vi "RVTBOX SampleCode_MultPort.vi"(11 "Modbus TCP Setting":T4={"TCP address"="192.168.178.2", "CH"=enum."Port1", "Sample Rate"=7812, "Port"=502}) -> ()   [LabVIEW 2022 SP3]
uses:
  Ctl/TCP Setting.ctl
  Ctl/Modbus Function TCP.ctl
  PortStatus.ctl
  E:/RVT_CONTROLBOX/RVT BOX SampleCode/LabVIEW/BOX SampleCode/DLL/Modbus.dll
  DLL/Modbus.dll
panel:
  in  "ON (Port1 ~ Port4) 2":bool[](array[boolean])=[TRUE, TRUE, FALSE, FALSE]
  out "Data Length 抓資料後的剩餘長度 2":u16(graph)=22989
  out "Waveform Chart 2":dbl[][](graph)=[[-0.00146484375, 0.0020751953125, -0.00146484375], [-0.000732421875, 0.001953125, -0.00048828125], [-0.00048828125, 0.000732421875, 0.0001220703125], [-0.001220703125, 0.0, 0.00048828125], [-0.002197265625, 0.001220703125, 0.0006103515625], [-0.002685546875, 0.0025634765625, 0.000732421875], [-0.0023193359375, 0.0018310546875, 0.0010986328125], [-0.0015869140625, 0.000732421875, 0.001708984375], [-0.001220703125, 0.000732421875, 0.002197265625], [-0.0018310546875, 0.0006103515625, 0.0020751953125], [-0.00244140625, -0.0003662109375, 0.0020751953125], [-0.0023193359375, -0.0006103515625, 0.0025634765625], [-0.002197265625, 0.00048828125, 0.0025634765625], [-0.0023193359375, 0.0009765625, 0.001953125], [-0.002197265625, 0.0003662109375, 0.0015869140625], [-0.0013427734375, 0.0003662109375, 0.0018310546875], [-0.0001220703125, 0.0006103515625, 0.0020751953125], [0.00048828125, 0.0001220703125, 0.0020751953125], [0.00048828125, 0.0, 0.001708984375], [0.0001220703125, 0.0009765625, 0.0013427734375], [0.0, 0.001708984375, 0.0010986328125], [-0.0001220703125, 0.0009765625, 0.0006103515625], [-0.0003662109375, 0.0, 0.0], [-0.0003662109375, 0.0, 0.0], [0.0, 0.0, 0.00048828125], [0.0003662109375, -0.00048828125, 0.00048828125], [0.0006103515625, -0.0009765625, 0.0001220703125], [0.0008544921875, -0.0006103515625, 0.000732421875], [0.000732421875, 0.0006103515625, 0.001708984375], [0.0003662109375, 0.002197265625, 0.0013427734375], [0.0001220703125, 0.003173828125, -0.000244140625], [0.0, 0.0029296875, -0.0013427734375], [-0.0010986328125, 0.00146484375, -0.0009765625], [-0.00244140625, 0.00048828125, 0.00048828125], [-0.002685546875, 0.000732421875, 0.0013427734375], [-0.00244140625, 0.0015869140625, 0.0008544921875], [-0.0015869140625, 0.0015869140625, 0.0001220703125], [-0.0006103515625, 0.00048828125, 0.0008544921875], [-0.00048828125, 0.0, 0.00146484375], [-0.001708984375, 0.0006103515625, 0.00048828125], [-0.001953125, 0.0008544921875, -0.000732421875], [-0.0006103515625, 0.0, -0.0001220703125], [0.0, -0.0003662109375, 0.0009765625], [-0.001220703125, 0.0003662109375, 0.0009765625], [-0.001953125, 0.0008544921875, 0.00048828125], [-0.0006103515625, 0.0006103515625, 0.00146484375], [0.0003662109375, 0.0006103515625, 0.003173828125], [-0.0003662109375, 0.0010986328125, 0.003662109375], [-0.001220703125, 0.0013427734375, 0.00244140625], [-0.001220703125, 0.0009765625, 0.00146484375], [-0.001708984375, 0.0, 0.001953125], [-0.002685546875, -0.001220703125, 0.00244140625], [-0.0029296875, -0.0010986328125, 0.0015869140625], [-0.0023193359375, 0.00048828125, 0.0003662109375], [-0.001708984375, 0.0013427734375, 0.000244140625], [-0.0010986328125, 0.0003662109375, 0.0009765625], [-0.0009765625, -0.000732421875, 0.0015869140625], [-0.001220703125, -0.0003662109375, 0.001708984375], [-0.000732421875, 0.0001220703125, 0.0006103515625], [-0.0001220703125, 0.0, -0.0009765625], [-0.00048828125, -0.00048828125, -0.0009765625], [-0.001220703125, -0.0003662109375, 0.0010986328125], [-0.000732421875, 0.0, 0.0025634765625], [0.0003662109375, 0.0003662109375, 0.0013427734375], [0.0010986328125, 0.000732421875, 0.0], [0.0013427734375, 0.0006103515625, 0.0], [0.0009765625, 0.00048828125, 0.0], [0.0, 0.0009765625, -0.0008544921875], [-0.0010986328125, 0.0018310546875, -0.001220703125], [-0.001708984375, 0.00146484375, -0.000244140625], [-0.0020751953125, 0.0001220703125, 0.0003662109375], [-0.0025634765625, -0.0001220703125, 0.00048828125], [-0.002197265625, 0.0003662109375, 0.00048828125], [-0.0010986328125, 0.000244140625, 0.000244140625], [-0.0003662109375, -0.0003662109375, -0.00048828125], [-0.000244140625, -0.0003662109375, -0.0010986328125], [-0.000244140625, 0.00048828125, -0.0009765625], [0.0, 0.0006103515625, -0.0009765625], [0.00048828125, 0.0, -0.0010986328125], [0.0008544921875, -0.0006103515625, -0.0001220703125], [0.0006103515625, -0.000732421875, 0.001220703125], [-0.0001220703125, -0.0010986328125, 0.001220703125], [-0.000732421875, -0.0006103515625, -0.0003662109375], [-0.0006103515625, 0.0008544921875, -0.0018310546875], [-0.0008544921875, 0.001953125, -0.001953125], [-0.0018310546875, 0.0015869140625, -0.001708984375], [-0.0025634765625, 0.000244140625, -0.0013427734375], [-0.002197265625, -0.0006103515625, -0.000732421875], [-0.0015869140625, -0.00146484375, 0.0], [-0.00146484375, -0.001708984375, 0.0006103515625], [-0.001220703125, -0.0010986328125, 0.0018310546875], [-0.0009765625, -0.0003662109375, 0.00244140625], [-0.001220703125, -0.0006103515625, 0.0013427734375], [-0.0018310546875, -0.0010986328125, 0.0], [-0.001953125, -0.000732421875, 0.0003662109375], [-0.001708984375, -0.0001220703125, 0.0018310546875], [-0.0018310546875, -0.0008544921875, 0.0020751953125], [-0.0015869140625, -0.001953125, 0.0010986328125], [-0.0003662109375, -0.001708984375, 0.0006103515625], [0.000244140625, -0.000244140625, 0.0008544921875], [-0.0003662109375, 0.000244140625, 0.0008544921875], [-0.0018310546875, -0.000244140625, 0.0001220703125], [-0.0020751953125, -0.000732421875, -0.0003662109375], [-0.0010986328125, -0.0003662109375, -0.000244140625], [-0.000244140625, 0.000244140625, 0.0], [-0.00048828125, 0.0, -0.000244140625], [-0.0010986328125, -0.0006103515625, -0.000732421875], [-0.0015869140625, -0.0009765625, -0.000244140625], [-0.001953125, -0.0006103515625, 0.0001220703125], [-0.0018310546875, -0.0003662109375, -0.000244140625], [-0.001220703125, -0.0003662109375, -0.000732421875], [-0.0009765625, -0.0001220703125, -0.0006103515625], [-0.0009765625, 0.0006103515625, -0.0006103515625], [-0.00048828125, 0.000732421875, -0.00048828125], [0.0006103515625, -0.000244140625, 0.000732421875], [0.0013427734375, -0.001220703125, 0.0015869140625], [0.0010986328125, -0.0006103515625, 0.0], [0.001220703125, 0.00048828125, -0.001953125], [0.001708984375, 0.0010986328125, -0.0018310546875], [0.000732421875, 0.0008544921875, -0.0008544921875], [-0.0015869140625, 0.0001220703125, -0.001220703125], [-0.003173828125, -0.0006103515625, -0.00146484375], [-0.0030517578125, -0.0006103515625, -0.000732421875], [-0.0023193359375, -0.000244140625, -0.000732421875], [-0.0015869140625, -0.001220703125, -0.0015869140625], [-0.000732421875, -0.0025634765625, -0.001220703125], [-0.0006103515625, -0.002197265625, 0.0], [-0.001220703125, -0.0008544921875, -0.0001220703125], [-0.0013427734375, -0.0006103515625, -0.000732421875], [-0.0003662109375, -0.0008544921875, -0.0003662109375], [0.0, 0.0, 0.0], [-0.0008544921875, 0.000732421875, -0.00048828125], [-0.001708984375, 0.0, -0.0006103515625], [-0.0018310546875, -0.0013427734375, 0.0001220703125], [-0.0015869140625, -0.001708984375, 0.0], [-0.000732421875, -0.00146484375, -0.0015869140625], [0.000244140625, -0.0015869140625, -0.001953125], [0.0003662109375, -0.0018310546875, -0.0008544921875], [-0.001220703125, -0.0018310546875, -0.0010986328125], [-0.0025634765625, -0.0013427734375, -0.00244140625], [-0.002197265625, -0.0010986328125, -0.0015869140625], [-0.0013427734375, -0.00146484375, 0.0008544921875], [-0.0018310546875, -0.0018310546875, 0.0013427734375], [-0.0020751953125, -0.0013427734375, -0.000244140625], [-0.0013427734375, -0.0006103515625, -0.0008544921875], [-0.0008544921875, -0.00048828125, 0.0], [-0.0008544921875, -0.00048828125, 0.0003662109375], [-0.000244140625, -0.0001220703125, -0.0001220703125], [0.000244140625, -0.00048828125, -0.00048828125], [-0.000244140625, -0.0015869140625, -0.000244140625], [-0.0006103515625, -0.00146484375, -0.0001220703125], [0.0001220703125, -0.000244140625, 0.0], [0.0008544921875, 0.0009765625, 0.0], [0.0006103515625, 0.0010986328125, 0.0003662109375], [0.0003662109375, 0.0001220703125, 0.000732421875], [0.0, -0.0009765625, 0.0009765625], [-0.000244140625, -0.0010986328125, 0.0009765625], [-0.0001220703125, 0.0, 0.0013427734375], [0.000732421875, 0.0, 0.0020751953125], [0.0006103515625, -0.001220703125, 0.001953125], [-0.0003662109375, -0.0020751953125, 0.0009765625], [-0.000732421875, -0.0009765625, 0.00048828125], [-0.0003662109375, 0.000244140625, 0.00146484375], [-0.000244140625, 0.000244140625, 0.00244140625], [-0.000244140625, -0.0003662109375, 0.001953125], [0.0001220703125, -0.0003662109375, 0.0013427734375], [0.000732421875, 0.0, 0.001708984375], [0.0013427734375, -0.000244140625, 0.00244140625], [0.0023193359375, -0.001220703125, 0.0028076171875], [0.001953125, -0.0010986328125, 0.0030517578125], [0.0, 0.0001220703125, 0.003173828125], [-0.001708984375, 0.0003662109375, 0.0028076171875], [-0.00146484375, -0.0010986328125, 0.00146484375], [-0.0008544921875, -0.001953125, 0.000244140625], [-0.00146484375, -0.00048828125, 0.0], [-0.00146484375, 0.000732421875, 0.0006103515625], [0.0001220703125, 0.00048828125, 0.0009765625], [0.001708984375, 0.00048828125, 0.0001220703125], [0.00146484375, 0.0013427734375, -0.00048828125], [0.0006103515625, 0.00146484375, 0.0003662109375], [0.0003662109375, 0.000244140625, 0.001953125], [-0.0001220703125, -0.0010986328125, 0.00146484375], [-0.00146484375, -0.002197265625, 0.0], [-0.001953125, -0.00244140625, -0.0001220703125], [-0.0008544921875, -0.0015869140625, 0.0008544921875], [0.000732421875, 0.0, 0.000732421875], [0.0018310546875, 0.0010986328125, -0.000244140625], [0.0023193359375, 0.000732421875, -0.000244140625], [0.00244140625, 0.0, 0.0003662109375], [0.002197265625, -0.0006103515625, 0.0], [0.0009765625, -0.001220703125, -0.0006103515625], [-0.001220703125, -0.001708984375, 0.0], [-0.0029296875, -0.001220703125, 0.0013427734375], [-0.002685546875, -0.0006103515625, 0.001708984375], [-0.0008544921875, -0.0009765625, 0.001220703125], [0.0006103515625, -0.00146484375, 0.000732421875], [0.001220703125, -0.000732421875, 0.0003662109375], [0.00146484375, 0.0006103515625, 0.0001220703125], [0.0009765625, 0.0006103515625, 0.000244140625], [0.0, -0.000244140625, 0.000244140625], [-0.0009765625, -0.0003662109375, 0.0], [-0.0010986328125, -0.00048828125, -0.0001220703125], [-0.0009765625, -0.0013427734375, -0.0001220703125], [-0.00146484375, -0.001708984375, 0.0006103515625], [-0.0015869140625, -0.0006103515625, 0.0020751953125], [-0.000732421875, 0.0003662109375, 0.0023193359375], [0.00048828125, 0.0, 0.000732421875], [0.0010986328125, -0.0001220703125, -0.0003662109375], [0.0009765625, -0.0001220703125, 0.000244140625], [0.0001220703125, -0.0008544921875, 0.0015869140625], [-0.0006103515625, -0.0015869140625, 0.001953125], [-0.0008544921875, -0.0015869140625, 0.001708984375], [-0.0003662109375, -0.001220703125, 0.001953125], [-0.0001220703125, -0.00048828125, 0.0020751953125], [0.0, 0.0003662109375, 0.0009765625], [0.00048828125, 0.0006103515625, -0.000244140625], [0.0008544921875, 0.0, -0.000244140625], [0.0008544921875, -0.0001220703125, 0.000244140625], [0.0010986328125, 0.0001220703125, 0.0], [0.001708984375, -0.0001220703125, -0.0006103515625], [0.00146484375, -0.0010986328125, -0.000244140625], [0.0001220703125, -0.0020751953125, 0.0006103515625], [-0.0010986328125, -0.0028076171875, 0.0006103515625], [-0.0018310546875, -0.002197265625, -0.0001220703125], [-0.0018310546875, 0.0, -0.0003662109375], [-0.0013427734375, 0.0008544921875, 0.0003662109375], [-0.00048828125, 0.0001220703125, 0.001220703125], [0.0, 0.0, 0.0010986328125], [-0.0001220703125, 0.0010986328125, 0.0003662109375], [0.0, 0.0015869140625, -0.0001220703125], [0.00048828125, 0.0013427734375, -0.0006103515625], [0.000732421875, 0.0010986328125, -0.0015869140625], [0.0, 0.00048828125, -0.0020751953125], [-0.00048828125, -0.0001220703125, -0.001220703125], [0.0, 0.0, -0.000244140625], [0.0015869140625, 0.0003662109375, -0.000244140625], [0.0029296875, 0.0001220703125, -0.0006103515625], [0.0025634765625, 0.0001220703125, 0.0], [0.00146484375, 0.00146484375, 0.00048828125], [0.0015869140625, 0.001953125, -0.0003662109375], [0.0018310546875, 0.000732421875, -0.0008544921875], [0.0, -0.0003662109375, -0.0001220703125], [-0.002685546875, -0.000244140625, 0.0], [-0.0035400390625, 0.000244140625, -0.0015869140625], [-0.001708984375, 0.00048828125, -0.002197265625], [-0.0001220703125, 0.00048828125, -0.001220703125], [0.0, 0.0006103515625, -0.0009765625], [0.0003662109375, 0.001220703125, -0.0013427734375], [0.0013427734375, 0.00146484375, -0.0009765625], [0.0013427734375, 0.0003662109375, -0.0001220703125], [0.0006103515625, -0.001220703125, 0.0], [0.0, -0.0018310546875, -0.00048828125], [-0.0006103515625, -0.001708984375, -0.0009765625], [-0.00146484375, -0.0013427734375, -0.001220703125], [-0.00146484375, -0.0010986328125, -0.000732421875], [-0.0003662109375, -0.00048828125, 0.0009765625], [0.0006103515625, 0.000244140625, 0.002197265625], [0.001220703125, 0.000732421875, 0.001953125], [0.0020751953125, 0.0003662109375, 0.001220703125], [0.0025634765625, -0.0003662109375, 0.001220703125], [0.00146484375, -0.0009765625, 0.0009765625], [-0.0008544921875, -0.00146484375, -0.0003662109375], [-0.0028076171875, -0.0020751953125, -0.0020751953125], [-0.0029296875, -0.0020751953125, -0.001953125], [-0.0020751953125, -0.000732421875, -0.000244140625], [-0.0006103515625, 0.000244140625, 0.0006103515625], [0.0009765625, 0.00048828125, -0.0001220703125], [0.0023193359375, 0.0008544921875, -0.00146484375], [0.002685546875, 0.001708984375, -0.0008544921875], [0.001953125, 0.001708984375, 0.00146484375], [0.0008544921875, 0.0009765625, 0.0032958984375], [0.00048828125, 0.0, 0.00244140625], [0.0, -0.0008544921875, 0.0], [-0.0008544921875, -0.0010986328125, -0.0018310546875], [-0.0008544921875, 0.000244140625, -0.001708984375], [0.00048828125, 0.001220703125, -0.0010986328125], [0.001220703125, 0.000244140625, -0.000732421875], [0.0, -0.00048828125, -0.000732421875], [-0.0003662109375, 0.0003662109375, -0.0008544921875], [0.0008544921875, 0.00146484375, -0.0006103515625], [0.001220703125, 0.00048828125, 0.0001220703125], [-0.00048828125, -0.0001220703125, 0.0009765625], [-0.001953125, 0.000732421875, 0.00048828125], [-0.00146484375, 0.0018310546875, -0.000732421875], [-0.0006103515625, 0.0015869140625, -0.00146484375], [-0.0008544921875, 0.000732421875, -0.001220703125], [-0.0010986328125, 0.0003662109375, -0.0006103515625], [-0.00048828125, 0.000732421875, -0.0001220703125], [0.000244140625, 0.0010986328125, 0.0001220703125], [0.0009765625, 0.000244140625, 0.0], [0.001708984375, -0.001220703125, -0.000244140625], [0.0015869140625, -0.0018310546875, 0.0], [0.0, -0.001220703125, 0.0006103515625], [-0.001708984375, -0.0006103515625, 0.00048828125], [-0.0013427734375, 0.0, -0.000732421875], [0.000244140625, 0.000732421875, -0.0010986328125], [0.0009765625, 0.0013427734375, 0.0006103515625], [0.0001220703125, 0.0010986328125, 0.0020751953125], [-0.0003662109375, 0.0010986328125, 0.0009765625], [0.0001220703125, 0.0010986328125, 0.0], [0.0010986328125, 0.00048828125, 0.0009765625], [0.0010986328125, -0.000244140625, 0.0018310546875], [0.0, -0.0006103515625, 0.0009765625], [-0.0009765625, -0.00048828125, 0.0003662109375], [-0.0008544921875, 0.0001220703125, 0.000732421875], [-0.0006103515625, 0.00146484375, 0.000732421875], [-0.0009765625, 0.0025634765625, 0.0006103515625], [-0.0009765625, 0.00244140625, 0.0010986328125], [-0.0003662109375, 0.001708984375, 0.0006103515625], [0.000244140625, 0.0010986328125, -0.0006103515625], [0.0009765625, 0.00048828125, -0.000732421875], [0.0018310546875, -0.0001220703125, -0.0001220703125], [0.0018310546875, -0.00048828125, -0.0003662109375], [0.0006103515625, -0.000244140625, 0.0], [-0.0008544921875, 0.0, 0.00146484375], [-0.0015869140625, 0.00048828125, 0.0018310546875], [-0.001220703125, 0.0015869140625, 0.0008544921875], [-0.00048828125, 0.00244140625, 0.0006103515625], [0.0001220703125, 0.0020751953125, 0.000732421875], [0.00048828125, 0.0006103515625, 0.0], [0.000732421875, 0.0, -0.000244140625], [0.0008544921875, 0.000244140625, 0.0006103515625], [0.000244140625, 0.000732421875, 0.00048828125], [-0.0010986328125, 0.000732421875, -0.0006103515625], [-0.0025634765625, 0.0006103515625, -0.0009765625], [-0.00341796875, 0.0009765625, -0.0006103515625], [-0.003173828125, 0.001708984375, -0.0008544921875], [-0.002197265625, 0.0020751953125, -0.00048828125], [-0.0010986328125, 0.001220703125, 0.0003662109375], [-0.000244140625, 0.0003662109375, 0.00048828125], [0.0, 0.00048828125, 0.0], [-0.001220703125, 0.0006103515625, -0.000244140625], [-0.00244140625, 0.0003662109375, -0.0001220703125], [-0.001708984375, 0.0003662109375, 0.0003662109375], [-0.0003662109375, 0.0006103515625, 0.001220703125], [-0.00048828125, 0.000732421875, 0.001708984375], [-0.001708984375, 0.000732421875, 0.0006103515625], [-0.00146484375, 0.0008544921875, -0.00048828125], [0.0, 0.000732421875, 0.0001220703125], [0.001220703125, 0.0006103515625, 0.002197265625], [0.0013427734375, 0.0010986328125, 0.002685546875], [0.000732421875, 0.00146484375, 0.00146484375], [-0.00048828125, 0.0006103515625, 0.0009765625], [-0.001708984375, 0.0, 0.0020751953125], [-0.002197265625, 0.000244140625, 0.002197265625], [-0.0015869140625, 0.0006103515625, 0.0006103515625], [-0.00048828125, 0.0, 0.0], [0.0001220703125, -0.00048828125, 0.0013427734375], [0.0001220703125, 0.0001220703125, 0.002197265625], [0.0, 0.0009765625, 0.001220703125], [0.00048828125, 0.0008544921875, 0.0008544921875], [0.001220703125, 0.0, 0.001708984375], [0.0009765625, -0.0009765625, 0.0015869140625], [0.0, -0.0010986328125, 0.0001220703125], [-0.000732421875, -0.0008544921875, -0.0003662109375], [-0.0009765625, -0.0009765625, 0.0], [-0.001220703125, -0.0010986328125, -0.0003662109375], [-0.0015869140625, 0.0001220703125, -0.001220703125], [-0.0015869140625, 0.0020751953125, -0.0009765625], [-0.0010986328125, 0.0029296875, 0.0], [-0.0003662109375, 0.0023193359375, 0.0], [0.0, 0.0020751953125, -0.00048828125], [0.000244140625, 0.002685546875, -0.0008544921875], [0.0010986328125, 0.0025634765625, -0.001220703125], [0.0010986328125, 0.0008544921875, -0.0023193359375], [0.0, -0.0003662109375, -0.0029296875], [-0.0013427734375, 0.0, -0.0018310546875], [-0.001953125, 0.0006103515625, 0.0], [-0.001953125, 0.00048828125, 0.0006103515625]]
  out "State":T3={"ControBoxState"=enum."BoxReady", "Port1"={"State"=enum."Bulk Mode", "PortOffset_Addr"=0, "Connected"=TRUE, "# samplesRVTbuffer"=22974}, "Port2"={"State"=enum."Bulk Mode", "PortOffset_Addr"=200, "Connected"=TRUE, "# samplesRVTbuffer"=22989}, "Port3"={"State"=enum."Reconnect Port", "PortOffset_Addr"=400, "Connected"=FALSE, "# samplesRVTbuffer"=0}, "Port4"={"State"=enum."Reconnect Port", "PortOffset_Addr"=600, "Connected"=FALSE, "# samplesRVTbuffer"=0}}
  out "Waveform Chart":dbl[][](graph)=[[0.002197265625, 0.0003662109375, 0.0], [0.000244140625, 0.0010986328125, -0.000244140625], [-0.00146484375, 0.001953125, -0.0006103515625], [0.0, 0.0008544921875, -0.000244140625], [0.0009765625, -0.000244140625, 0.0], [0.00048828125, 0.0001220703125, -0.0001220703125], [0.0, 0.000244140625, -0.0003662109375], [0.0001220703125, -0.0009765625, 0.0], [0.0008544921875, -0.001953125, 0.0006103515625], [0.0018310546875, -0.001708984375, 0.000244140625], [0.001220703125, -0.000732421875, -0.0001220703125], [0.00048828125, 0.0003662109375, 0.0003662109375], [0.001953125, 0.00048828125, 0.0009765625], [0.0023193359375, 0.0, 0.000732421875], [0.000244140625, 0.000244140625, 0.000732421875], [0.0, 0.000732421875, 0.0008544921875], [0.0015869140625, -0.000244140625, 0.000732421875], [0.001708984375, -0.0008544921875, 0.000732421875], [0.0010986328125, -0.0003662109375, 0.0009765625], [0.0018310546875, -0.0003662109375, 0.0003662109375], [0.002197265625, -0.0006103515625, 0.0], [0.0010986328125, -0.0001220703125, 0.0003662109375], [0.0003662109375, -0.0001220703125, 0.0006103515625], [0.0001220703125, -0.0008544921875, 0.000244140625], [0.0, -0.00048828125, 0.0001220703125], [0.0010986328125, 0.0003662109375, 0.0], [0.002685546875, 0.0, 0.0], [0.0029296875, -0.0009765625, 0.0006103515625], [0.0030517578125, -0.001220703125, 0.000732421875], [0.003173828125, -0.0008544921875, 0.000244140625], [0.001708984375, -0.00048828125, 0.000244140625], [-0.000244140625, -0.0001220703125, 0.0003662109375], [-0.000244140625, 0.0006103515625, 0.0], [0.001220703125, 0.0010986328125, -0.000244140625], [0.001953125, 0.0, -0.000244140625], [0.00146484375, -0.0015869140625, -0.0006103515625], [0.001220703125, -0.0018310546875, -0.0003662109375], [0.0015869140625, -0.0010986328125, 0.0001220703125], [0.0013427734375, -0.000732421875, 0.0003662109375], [0.000244140625, -0.0001220703125, 0.00048828125], [-0.0001220703125, 0.0003662109375, 0.0009765625], [0.0006103515625, -0.000244140625, 0.000732421875], [0.0010986328125, -0.001220703125, -0.0001220703125], [0.00048828125, -0.0006103515625, -0.0003662109375], [-0.000244140625, 0.0003662109375, 0.0003662109375], [-0.00048828125, 0.0, 0.0010986328125], [0.0, -0.00048828125, 0.0008544921875], [0.000732421875, 0.0001220703125, 0.000244140625], [0.0013427734375, 0.00048828125, 0.0], [0.0013427734375, -0.0009765625, 0.000244140625], [0.0006103515625, -0.0018310546875, 0.0009765625], [0.0, -0.00048828125, 0.001708984375], [0.0001220703125, 0.0010986328125, 0.0009765625], [0.0010986328125, 0.0008544921875, -0.0003662109375], [0.0015869140625, -0.0001220703125, -0.0001220703125], [0.00146484375, -0.00048828125, 0.0008544921875], [0.0010986328125, -0.0008544921875, 0.0010986328125], [0.0015869140625, -0.0013427734375, 0.000732421875], [0.003173828125, -0.0015869140625, 0.0006103515625], [0.0032958984375, -0.0013427734375, 0.0006103515625], [0.00048828125, -0.000732421875, 0.001220703125], [-0.00048828125, -0.000244140625, 0.001708984375], [0.001220703125, -0.0001220703125, 0.0013427734375], [0.001220703125, 0.0001220703125, 0.00146484375], [-0.000732421875, 0.0006103515625, 0.0020751953125], [-0.0006103515625, 0.000732421875, 0.0009765625], [0.0013427734375, 0.000244140625, -0.000244140625], [0.0020751953125, -0.0001220703125, 0.0003662109375], [0.0008544921875, -0.000244140625, 0.001220703125], [-0.0001220703125, -0.00048828125, 0.0003662109375], [0.0003662109375, -0.0008544921875, -0.0001220703125], [0.0010986328125, -0.0006103515625, 0.0006103515625], [-0.000732421875, -0.000244140625, 0.0013427734375], [-0.002197265625, -0.0006103515625, 0.0013427734375], [0.000244140625, -0.0009765625, 0.000732421875], [0.002685546875, 0.0, 0.0003662109375], [0.0018310546875, 0.000244140625, 0.000732421875], [0.0013427734375, -0.0003662109375, 0.0008544921875], [0.0020751953125, -0.0003662109375, 0.0001220703125], [0.00146484375, 0.0003662109375, -0.0003662109375], [0.000732421875, 0.0001220703125, 0.0], [0.0013427734375, 0.0, 0.0006103515625], [0.0009765625, 0.0010986328125, 0.0010986328125], [0.0, 0.001220703125, 0.0008544921875], [0.000732421875, -0.0001220703125, -0.0003662109375], [0.0025634765625, -0.0010986328125, -0.0015869140625], [0.003173828125, -0.000732421875, -0.00146484375], [0.0018310546875, 0.0001220703125, -0.000732421875], [0.0008544921875, -0.0001220703125, -0.0001220703125], [0.0020751953125, -0.00146484375, 0.0001220703125], [0.0028076171875, -0.001220703125, 0.00048828125], [0.0013427734375, 0.000732421875, 0.00048828125], [0.0009765625, 0.0013427734375, 0.0], [0.0020751953125, 0.0, 0.0], [0.0020751953125, -0.0003662109375, 0.0003662109375], [0.001220703125, -0.000244140625, 0.000244140625], [0.0013427734375, -0.0009765625, -0.000244140625], [0.0010986328125, -0.0010986328125, -0.0006103515625], [0.0008544921875, -0.0001220703125, 0.0], [0.001953125, -0.000244140625, 0.0003662109375], [0.002197265625, -0.0009765625, 0.0001220703125], [0.0006103515625, -0.0006103515625, -0.0006103515625], [0.0003662109375, -0.0001220703125, -0.0006103515625], [0.0008544921875, -0.000244140625, 0.0], [-0.00048828125, -0.000244140625, 0.0003662109375], [-0.0015869140625, 0.0001220703125, 0.0006103515625], [0.0006103515625, 0.0003662109375, 0.0009765625], [0.003662109375, -0.00048828125, 0.00146484375], [0.0029296875, -0.0020751953125, 0.00146484375], [0.0001220703125, -0.0028076171875, 0.000732421875], [0.0, -0.001708984375, 0.0], [0.001953125, -0.00048828125, 0.0], [0.001220703125, 0.000244140625, -0.000244140625], [-0.001220703125, 0.0006103515625, -0.0009765625], [-0.0009765625, 0.000244140625, -0.000732421875], [0.0018310546875, -0.00048828125, 0.00048828125], [0.0023193359375, -0.000732421875, 0.0008544921875], [0.0, -0.000244140625, -0.0001220703125], [-0.0003662109375, -0.000244140625, -0.0008544921875], [0.001708984375, -0.00048828125, -0.001220703125], [0.0025634765625, -0.0001220703125, -0.0013427734375], [0.000732421875, 0.0001220703125, -0.000244140625], [0.00048828125, -0.0001220703125, 0.0010986328125], [0.002685546875, -0.0008544921875, 0.0009765625], [0.0028076171875, -0.001220703125, 0.0], [0.000244140625, -0.0009765625, 0.0001220703125], [-0.001220703125, -0.0001220703125, 0.0009765625], [0.0, 0.0001220703125, 0.0013427734375], [0.001953125, -0.0008544921875, 0.001220703125], [0.0015869140625, -0.0018310546875, 0.0013427734375], [-0.0006103515625, -0.001708984375, 0.00146484375], [-0.0003662109375, -0.00146484375, 0.0009765625], [0.002197265625, -0.00146484375, 0.0001220703125], [0.001708984375, -0.0006103515625, 0.0003662109375], [-0.0010986328125, 0.000244140625, 0.0006103515625], [0.0, -0.0009765625, 0.0], [0.0029296875, -0.0032958984375, -0.000244140625], [0.0015869140625, -0.0030517578125, 0.0003662109375], [-0.0008544921875, -0.00048828125, 0.0003662109375], [0.0006103515625, 0.0, -0.00048828125], [0.0028076171875, -0.00146484375, -0.000732421875], [0.0018310546875, -0.001708984375, 0.0001220703125], [0.0003662109375, 0.0, 0.0006103515625], [0.0009765625, 0.0, 0.000244140625], [0.001708984375, -0.001220703125, 0.0003662109375], [0.0001220703125, -0.001220703125, 0.000732421875], [-0.0009765625, -0.0003662109375, 0.0006103515625], [0.000732421875, -0.0008544921875, 0.00048828125], [0.0023193359375, -0.001708984375, 0.000732421875], [-0.000244140625, -0.0008544921875, 0.0008544921875], [-0.00244140625, 0.0, 0.0003662109375], [0.000732421875, -0.0009765625, 0.0], [0.00341796875, -0.0023193359375, -0.0003662109375], [0.0010986328125, -0.0015869140625, -0.0006103515625], [-0.0006103515625, -0.0001220703125, -0.000732421875], [0.0008544921875, 0.000244140625, -0.0006103515625], [0.0008544921875, 0.000732421875, -0.0003662109375], [-0.0015869140625, 0.0009765625, -0.000244140625], [-0.0018310546875, 0.000244140625, -0.000732421875], [0.000732421875, 0.0, -0.00048828125], [0.0025634765625, 0.000732421875, 0.000732421875], [0.00146484375, 0.000732421875, 0.0008544921875], [-0.000244140625, 0.0001220703125, -0.0006103515625], [-0.0001220703125, 0.00048828125, -0.000732421875], [0.00146484375, 0.0008544921875, 0.000732421875], [0.0018310546875, 0.0008544921875, 0.0008544921875], [0.000732421875, 0.0013427734375, -0.000244140625], [0.00048828125, 0.0013427734375, -0.000244140625], [0.0008544921875, 0.0001220703125, 0.0006103515625], [0.0010986328125, -0.0001220703125, 0.00048828125], [0.000244140625, 0.001220703125, -0.000244140625], [-0.0018310546875, 0.0018310546875, -0.0008544921875], [-0.00244140625, 0.0006103515625, -0.0009765625], [0.0001220703125, 0.0, -0.000732421875], [0.001220703125, 0.000244140625, -0.000244140625], [-0.0008544921875, 0.0003662109375, -0.0001220703125], [-0.000244140625, -0.000244140625, -0.0009765625], [0.0023193359375, -0.000244140625, -0.0010986328125], [0.0009765625, 0.001220703125, -0.000244140625], [-0.0010986328125, 0.001708984375, -0.00048828125], [0.000732421875, 0.00048828125, -0.001220703125], [0.0025634765625, -0.000244140625, -0.0001220703125], [0.0015869140625, -0.0003662109375, 0.0006103515625], [0.001953125, -0.000732421875, -0.00048828125], [0.0030517578125, -0.000732421875, -0.0003662109375], [0.001220703125, -0.000244140625, 0.0013427734375], [-0.0020751953125, 0.0003662109375, 0.000244140625], [-0.00341796875, 0.0020751953125, -0.001708984375], [-0.0020751953125, 0.003173828125, -0.000244140625], [0.0001220703125, 0.001953125, 0.0010986328125], [0.0006103515625, 0.00048828125, -0.0001220703125], [0.000244140625, 0.0001220703125, -0.0003662109375], [0.0010986328125, -0.0010986328125, 0.0008544921875], [0.0013427734375, -0.0018310546875, 0.0006103515625], [0.0, 0.0, -0.0001220703125], [0.0001220703125, 0.002197265625, 0.0], [0.0008544921875, 0.0020751953125, -0.0001220703125], [0.0, 0.00146484375, -0.000732421875], [-0.0003662109375, 0.0013427734375, -0.0006103515625], [0.0009765625, 0.00048828125, 0.0], [0.000732421875, 0.0001220703125, 0.000244140625], [-0.0008544921875, 0.0009765625, -0.0003662109375], [-0.001708984375, 0.001708984375, -0.0013427734375], [-0.001220703125, 0.0010986328125, -0.0009765625], [0.000732421875, 0.0, -0.000732421875], [0.002197265625, 0.0006103515625, -0.0009765625], [0.0006103515625, 0.001953125, -0.000244140625], [-0.0001220703125, 0.0006103515625, 0.000732421875], [0.0020751953125, -0.0013427734375, -0.0003662109375], [0.001708984375, 0.0, -0.00146484375], [-0.001220703125, 0.0025634765625, -0.0008544921875], [-0.001220703125, 0.0020751953125, -0.00048828125], [0.0, 0.0008544921875, -0.0008544921875], [-0.0009765625, 0.0015869140625, -0.00048828125], [-0.0010986328125, 0.0020751953125, -0.0001220703125], [0.0001220703125, 0.00146484375, -0.00048828125], [-0.0003662109375, 0.0015869140625, 0.0], [-0.0006103515625, 0.00146484375, 0.0], [0.001220703125, 0.0, -0.0006103515625], [0.0015869140625, -0.0008544921875, -0.0003662109375], [-0.000244140625, 0.0001220703125, 0.0003662109375], [-0.000732421875, 0.000732421875, 0.000244140625], [0.0003662109375, 0.0003662109375, -0.0003662109375], [0.0009765625, 0.0003662109375, -0.0006103515625], [0.000244140625, 0.0006103515625, -0.0008544921875], [-0.0010986328125, 0.0, -0.0006103515625], [-0.001708984375, -0.00048828125, -0.0001220703125], [-0.0003662109375, -0.0006103515625, -0.0003662109375], [0.000732421875, -0.0006103515625, -0.0008544921875], [0.0, -0.00048828125, -0.0008544921875], [-0.0010986328125, 0.0, -0.00048828125], [-0.001708984375, 0.000732421875, 0.0], [-0.00244140625, 0.0013427734375, 0.0], [-0.0020751953125, 0.0013427734375, -0.0003662109375], [-0.0003662109375, 0.0001220703125, -0.000244140625], [0.0, -0.00048828125, 0.0003662109375], [-0.000732421875, 0.0003662109375, -0.0001220703125], [-0.000732421875, 0.001220703125, -0.0010986328125], [-0.001220703125, 0.0010986328125, 0.0], [-0.0029296875, 0.001220703125, 0.0013427734375], [-0.002685546875, 0.0015869140625, 0.0003662109375], [-0.000244140625, 0.001708984375, -0.0008544921875], [0.0, 0.0015869140625, -0.00048828125], [-0.0013427734375, 0.001220703125, 0.0], [-0.0010986328125, 0.001220703125, -0.000732421875], [0.00048828125, 0.002197265625, -0.00048828125], [-0.00048828125, 0.002685546875, 0.0006103515625], [-0.0028076171875, 0.001953125, 0.0009765625], [-0.00146484375, 0.001220703125, 0.0009765625], [0.0009765625, 0.0010986328125, 0.0010986328125], [-0.00048828125, 0.001220703125, 0.00048828125], [-0.0029296875, 0.0015869140625, -0.0001220703125], [-0.0006103515625, 0.00146484375, 0.0001220703125], [0.0018310546875, 0.0008544921875, 0.0006103515625], [-0.0003662109375, 0.0013427734375, 0.0], [-0.0020751953125, 0.0025634765625, -0.0001220703125], [0.0001220703125, 0.0028076171875, 0.0001220703125], [0.0023193359375, 0.00244140625, 0.0], [0.0018310546875, 0.0015869140625, -0.00048828125], [0.0009765625, 0.00048828125, -0.0008544921875], [0.0006103515625, 0.000244140625, -0.0009765625], [0.0010986328125, 0.001220703125, -0.0010986328125], [0.000732421875, 0.0023193359375, -0.0006103515625], [-0.0015869140625, 0.0030517578125, 0.0001220703125], [-0.001953125, 0.0032958984375, 0.0001220703125], [0.0006103515625, 0.0028076171875, -0.000732421875], [0.000244140625, 0.0029296875, -0.0006103515625], [-0.002685546875, 0.00341796875, 0.000244140625], [-0.00244140625, 0.0025634765625, -0.000244140625], [-0.000732421875, 0.00146484375, -0.0013427734375], [-0.001708984375, 0.001708984375, -0.000244140625], [-0.0028076171875, 0.0020751953125, 0.0009765625], [-0.001708984375, 0.0013427734375, 0.0], [-0.0008544921875, 0.0008544921875, -0.0009765625], [-0.0001220703125, 0.0009765625, -0.00048828125], [0.000732421875, 0.0006103515625, -0.0001220703125], [0.0006103515625, 0.0, -0.0009765625], [-0.0008544921875, 0.0008544921875, -0.0008544921875], [-0.00244140625, 0.002685546875, 0.0001220703125], [-0.0030517578125, 0.0028076171875, 0.0], [-0.001708984375, 0.0010986328125, -0.0008544921875], [0.000244140625, 0.0001220703125, -0.0003662109375], [0.000732421875, 0.0001220703125, 0.00048828125], [-0.0001220703125, -0.00048828125, 0.000244140625], [-0.000732421875, -0.001220703125, -0.000244140625], [-0.0003662109375, -0.0003662109375, -0.0003662109375], [-0.0008544921875, 0.0013427734375, -0.000732421875], [-0.002197265625, 0.00244140625, -0.000732421875], [-0.00146484375, 0.0015869140625, -0.000244140625], [0.0010986328125, -0.000732421875, -0.0008544921875], [0.0008544921875, -0.002197265625, -0.001220703125], [-0.0018310546875, -0.00146484375, 0.0], [-0.0023193359375, -0.000732421875, 0.000244140625], [-0.0010986328125, -0.000732421875, -0.001220703125], [-0.001708984375, -0.0001220703125, -0.0009765625], [-0.0018310546875, 0.0006103515625, 0.00048828125], [-0.000732421875, 0.0006103515625, 0.0003662109375], [-0.0009765625, 0.0010986328125, -0.00048828125], [-0.0009765625, 0.001220703125, -0.0006103515625], [0.000732421875, 0.0, -0.0008544921875], [-0.0001220703125, 0.000244140625, -0.00048828125], [-0.003173828125, 0.0015869140625, 0.0006103515625], [-0.0020751953125, 0.0008544921875, 0.000732421875], [0.00048828125, 0.0001220703125, 0.0], [-0.0006103515625, 0.00146484375, 0.0006103515625], [-0.0028076171875, 0.001708984375, 0.001220703125], [-0.002197265625, 0.00048828125, 0.0008544921875], [-0.001220703125, 0.0009765625, 0.000732421875], [-0.0023193359375, 0.0020751953125, 0.00048828125], [-0.0032958984375, 0.0008544921875, -0.000244140625], [-0.0018310546875, -0.0008544921875, -0.00048828125], [-0.000732421875, -0.0008544921875, 0.000244140625], [-0.0018310546875, 0.0, 0.00048828125], [-0.002197265625, 0.00048828125, 0.000732421875], [-0.0006103515625, 0.0003662109375, 0.0013427734375], [-0.0006103515625, 0.00048828125, 0.0008544921875], [-0.001953125, 0.001220703125, 0.000244140625], [-0.0010986328125, 0.001220703125, 0.0009765625], [-0.0006103515625, 0.0003662109375, 0.0015869140625], [-0.00244140625, 0.0, 0.000732421875], [-0.0020751953125, 0.0, 0.0], [0.0, 0.0, 0.0], [-0.00048828125, 0.000244140625, 0.0003662109375], [-0.0013427734375, 0.0003662109375, 0.000732421875], [0.0006103515625, 0.0001220703125, 0.000244140625], [0.0010986328125, 0.000244140625, -0.00048828125], [-0.0018310546875, 0.0009765625, -0.0003662109375], [-0.00244140625, 0.0013427734375, 0.0001220703125], [0.000244140625, 0.001708984375, 0.0001220703125], [0.0010986328125, 0.001708984375, 0.0001220703125], [-0.000244140625, 0.00146484375, 0.0009765625], [-0.0009765625, 0.001220703125, 0.001708984375], [-0.00048828125, 0.0008544921875, 0.0013427734375], [0.0, 0.0006103515625, 0.0001220703125], [0.0, 0.0008544921875, -0.0006103515625], [-0.000244140625, 0.0009765625, -0.000244140625], [-0.0003662109375, 0.0006103515625, 0.0003662109375], [-0.001220703125, 0.00048828125, 0.0], [-0.001220703125, 0.0009765625, -0.0008544921875], [0.000244140625, 0.0009765625, -0.00048828125], [0.0001220703125, 0.0009765625, 0.0001220703125], [-0.001953125, 0.0015869140625, -0.0001220703125], [-0.0015869140625, 0.0009765625, -0.0003662109375], [0.000732421875, -0.00048828125, 0.000244140625], [-0.000244140625, 0.0, 0.000244140625], [-0.0023193359375, 0.0018310546875, -0.000732421875], [-0.0008544921875, 0.001708984375, -0.0006103515625], [0.0003662109375, 0.00048828125, 0.000732421875], [-0.000732421875, 0.000244140625, 0.000732421875], [-0.0006103515625, 0.0001220703125, -0.0006103515625], [0.00048828125, 0.0001220703125, -0.0006103515625], [0.0, 0.001220703125, 0.00048828125], [-0.0001220703125, 0.00146484375, 0.000244140625], [0.00048828125, 0.0006103515625, -0.0003662109375], [0.0, 0.00048828125, 0.0003662109375], [-0.0003662109375, 0.0008544921875, 0.0006103515625], [0.0013427734375, -0.0003662109375, -0.00048828125], [0.0025634765625, -0.0013427734375, -0.000732421875], [0.0010986328125, -0.000244140625, -0.0001220703125], [-0.0008544921875, 0.0009765625, -0.00048828125], [-0.000732421875, 0.0008544921875, -0.00048828125], [0.0010986328125, 0.000244140625, 0.0], [0.0015869140625, 0.0, -0.000732421875], [0.0001220703125, 0.0001220703125, -0.0015869140625], [0.000244140625, 0.0, -0.000732421875], [0.0025634765625, -0.00048828125, 0.0008544921875], [0.0020751953125, -0.00048828125, 0.001220703125], [-0.0009765625, 0.0003662109375, 0.00048828125], [-0.001708984375, 0.0009765625, 0.0]]
  out "Failure  (Port1 ~ Port4)":bool[](array[boolean])
  out "Connted (Port1 ~ Port4)":bool[](array[boolean])=[TRUE, TRUE, FALSE, FALSE]
  out "Device ID":u16=1
  out "Stop Time":timestamp=timestamp(3855977902.205061 s since 1904-01-01)
  in  "stop":bool=TRUE
  out "Data Length 抓資料後的剩餘長度":u16(graph)=22974
  out "Iteration":i32=755
  out "Next #":u16=22974
  out "error out":errorcluster
  # "BOX只示範抓PORT1/2,有時會TIMEOUT,但會再回來續抓資料"
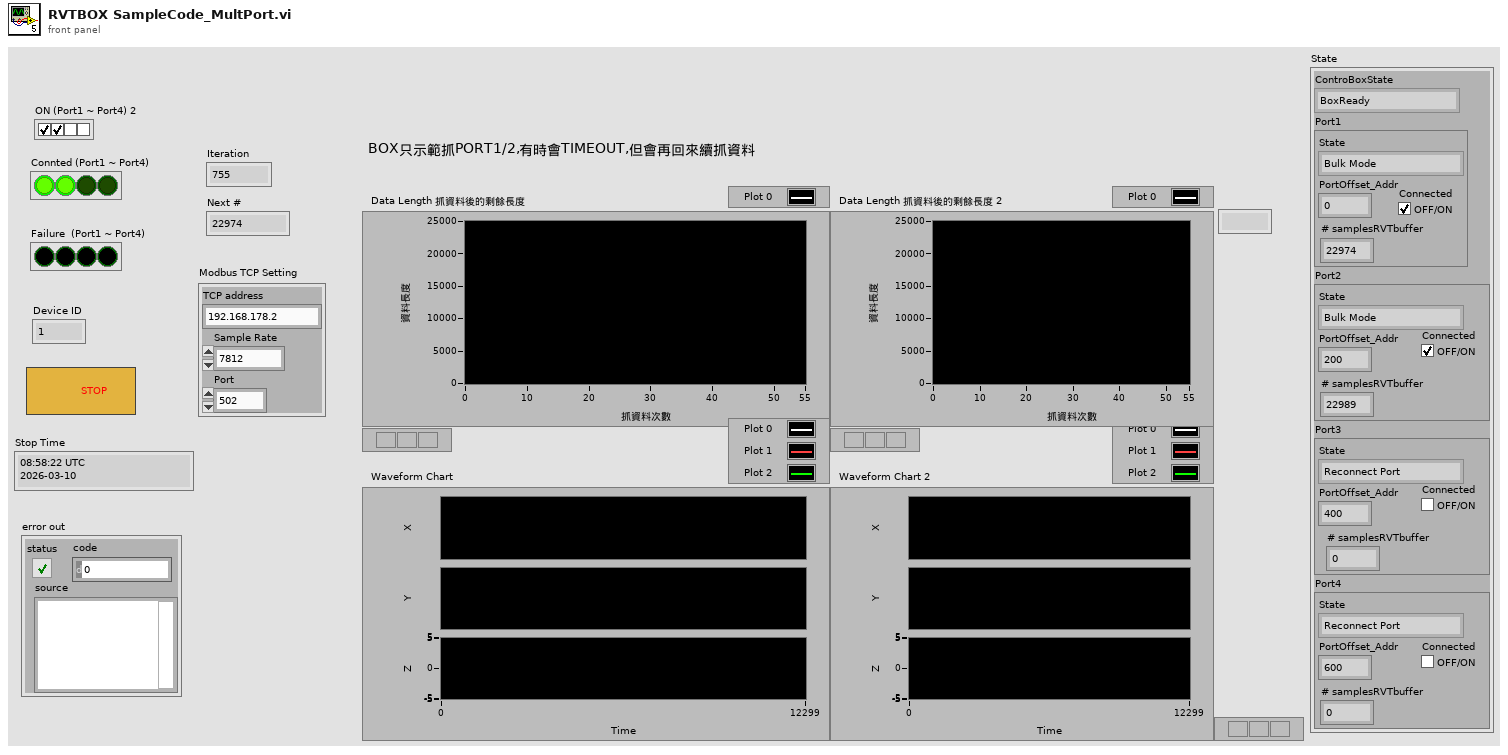
[diagram p1: front panel]
types:
  T1 = typedef "Modbus Function TCP.ctl" = enum16{"Get Data Length", "Normal Mode", "Bulk Mode", "Reconnect Port", "Recconect Box", "BoxReady"}
  T2 = typedef "PortStatus.ctl" = cluster{"State":T1, "PortOffset_Addr":u16, "Connected":bool, "# samplesRVTbuffer":u16}
  T3 = cluster{"ControBoxState":T1, "Port1":T2, "Port2":T2, "Port3":T2, "Port4":T2}
  T4 = typedef "TCP Setting.ctl" = cluster{"TCP address":string, "CH":enum16{"Port1", "Port2", "Port3", "Port4"}, "Sample Rate":u16, "Port":i32}
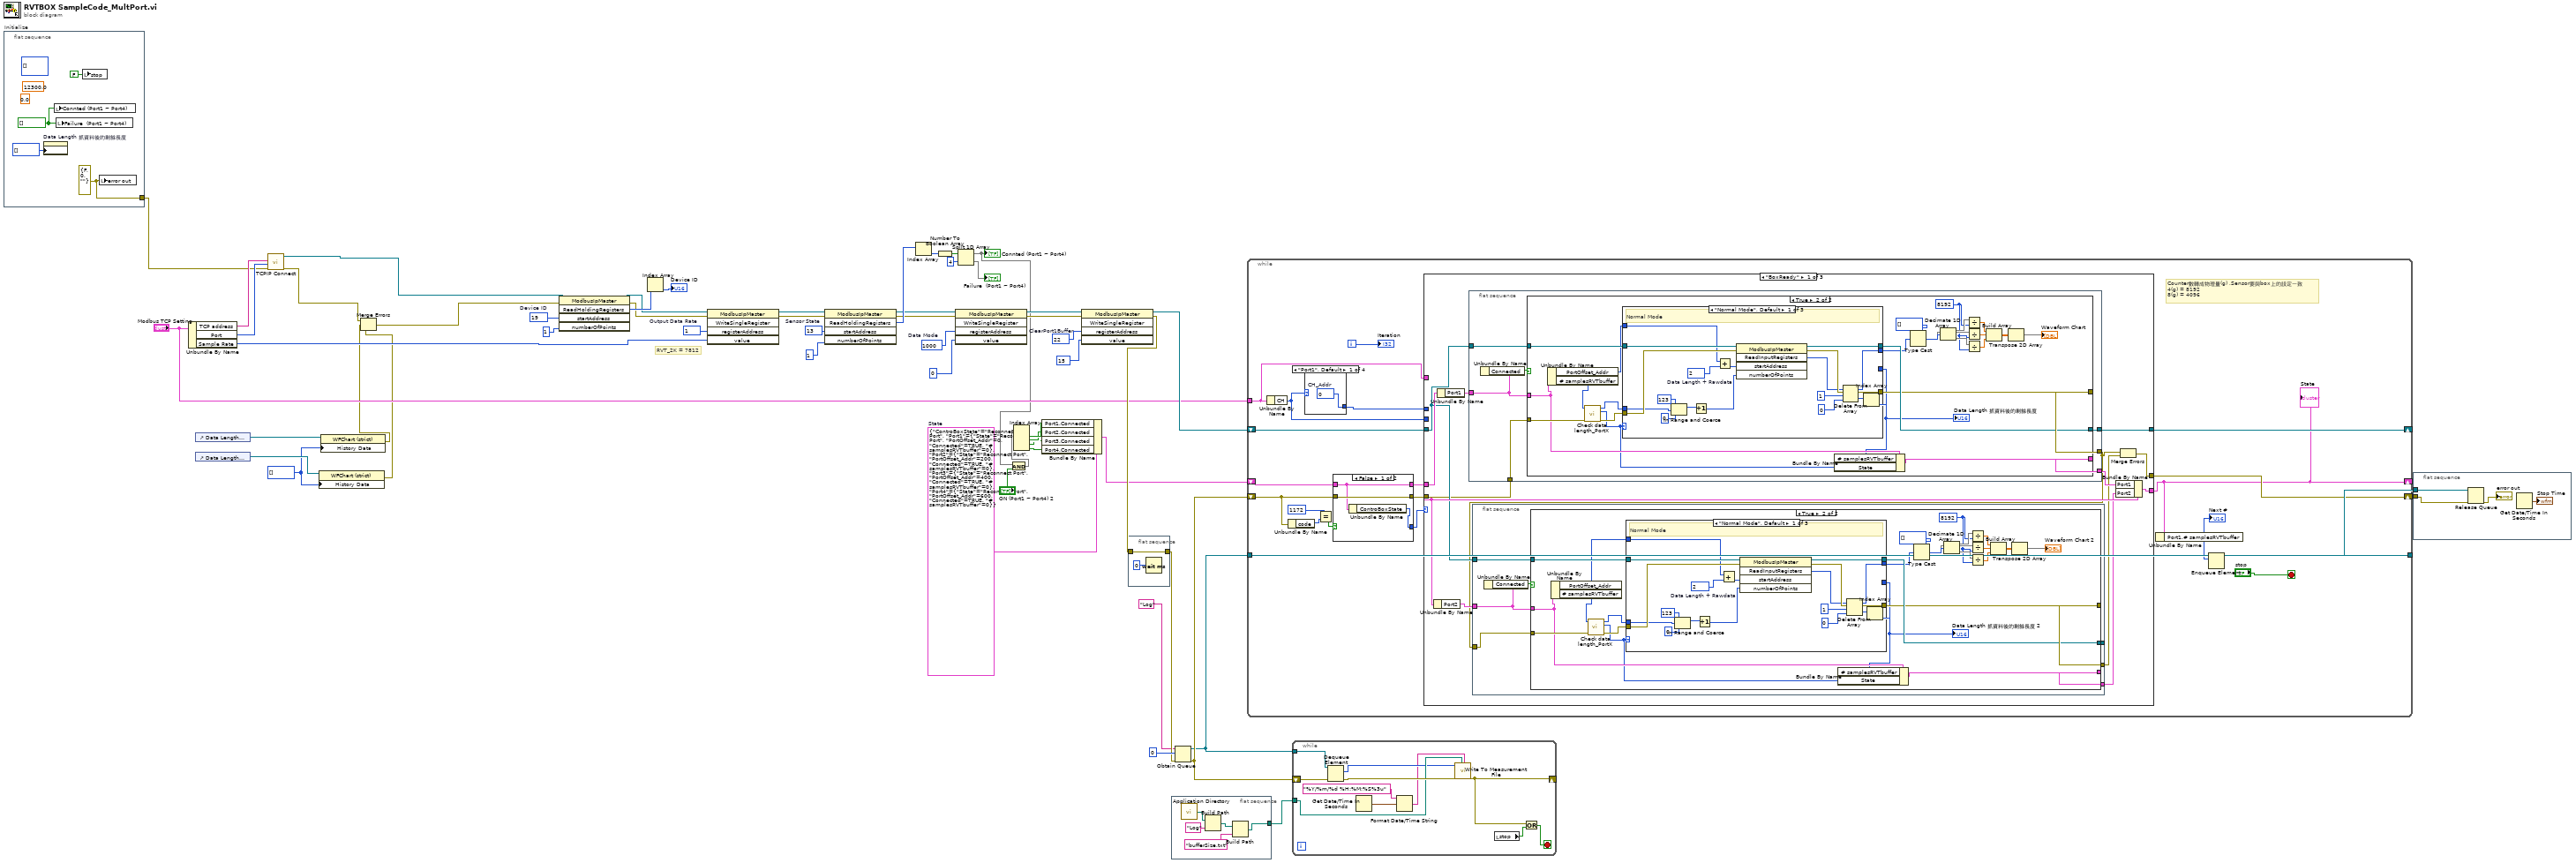
[diagram p0: block diagram]
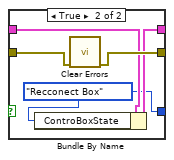
[diagram p2: hidden frame]
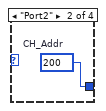
[diagram p3: hidden frame]
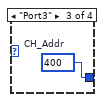
[diagram p4: hidden frame]
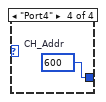
[diagram p5: hidden frame]
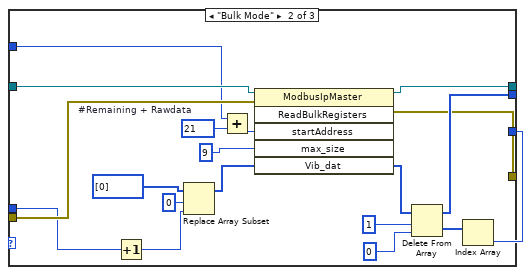
[diagram p7: hidden frame]
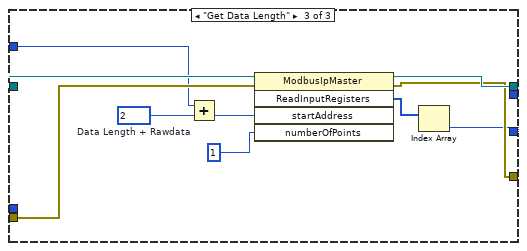
[diagram p8: hidden frame]
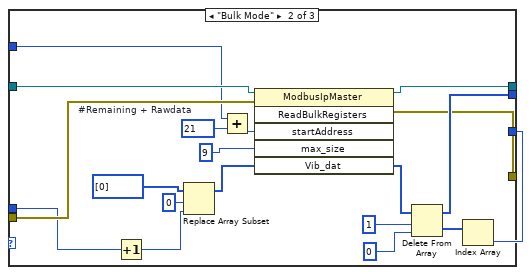
[diagram p10: hidden frame]
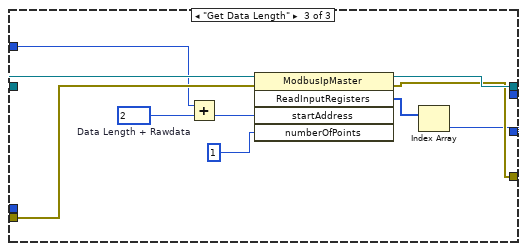
[diagram p11: hidden frame]
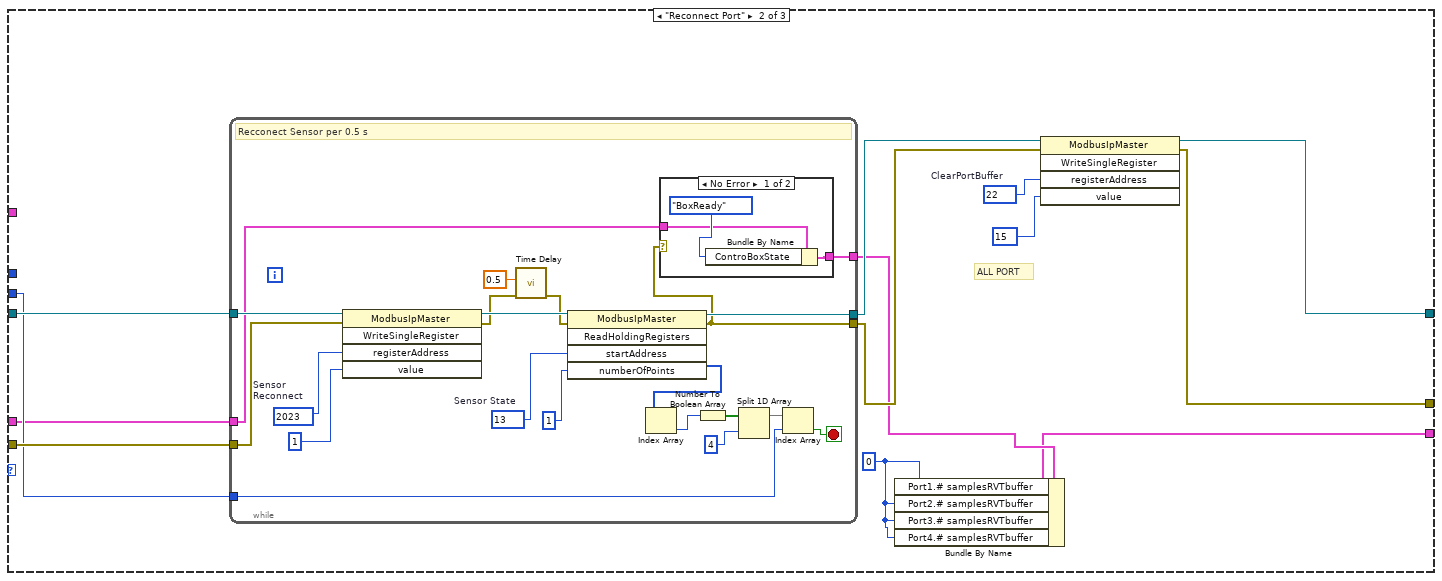
[diagram p12: hidden frame]
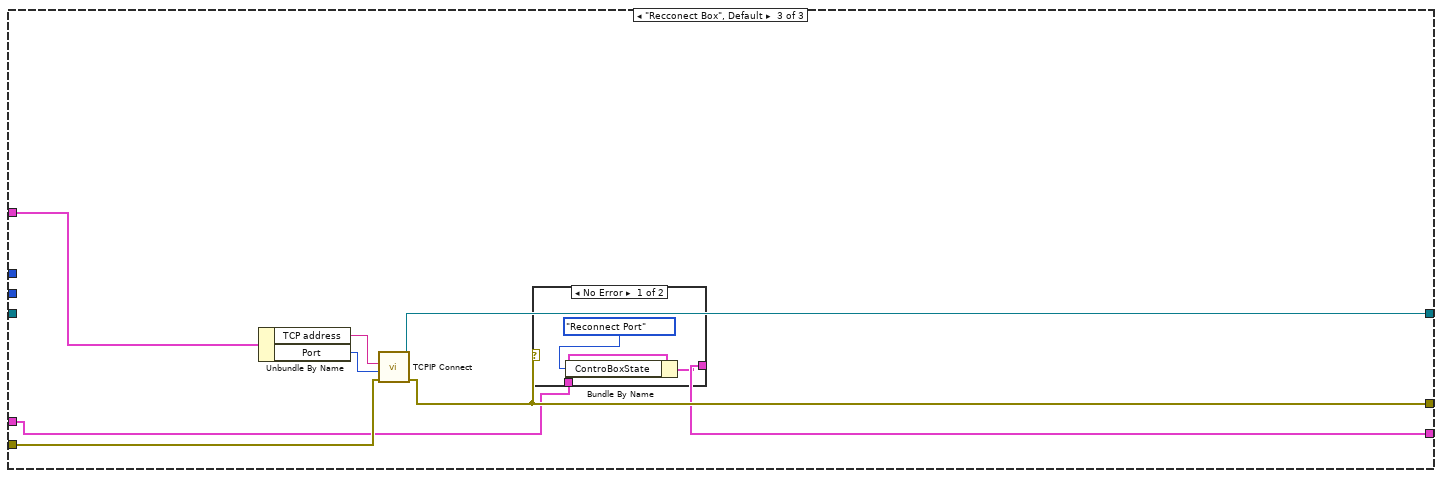
[diagram p14: hidden frame]
diagram:
  w4 = i32[] []
  w16 = T3 {"ControBoxState"=enum."Reconnect Port", "Port1"={"State"=enum."Reconnect Port", "PortOffset_Addr"=0, "Connected"=TRUE, "# samplesRVTbuffer"=0}, "Port2"={"State"=enum."Reconnect Port", "PortOffset_Addr"=200, "Connected"=TRUE, "# samplesRVTbuffer"=0}, "Port3"={"State"=enum."Reconnect Port", "PortOffset_Addr"=400, "Connected"=TRUE, "# samplesRVTbuffer"=0}, "Port4"={"State"=enum."Reconnect Port", "PortOffset_Addr"=600, "Connected"=TRUE, "# samplesRVTbuffer"=0}}  # State
  w30 = u16 1000  # Data Mode
  w33 = u16 22  # ClearPort1Buffer
  w42 = u16 13  # Sensor State
  w47 = u16 19  # Device ID
  w49 = u16 1  # Output Data Rate
  # "RVT_2K = 7812"
  n1 = flat-sequence "Initialize" {
    tunnel: [w60] -> w23
    frame #0 {
      (unwired) 12300.0 ("X Scale.Range:Maximum")
      (unwired) 0.0 ("X Scale.Range:Minimum")
      (unwired) i16[][] []
      w59 = bool[] [] ("Failure ? (Port1 ~ Port4)")
      w60 = errorcluster {"status"=FALSE, "code"=0, "source"=""} ("error out")
      n2 = property on="Data Length 抓資料後的剩餘長度" class="WFChart (strict)"("History Data"=u16[] []) -> ()  [unwired: 2 in, 2 out]
      n3 = local write "Connted (Port1 ~ Port4)"(w59) -> ()
      n4 = local write "Failure  (Port1 ~ Port4)"(w59) -> ()
      n5 = local write "stop"(FALSE ("stop")) -> ()
      n6 = local write "error out"(w60) -> ()
    }
  }
  n7 = Unbundle By Name("Modbus TCP Setting") -> ("TCP address"=w25:string, "Port"=w24:i32, "Sample Rate"=w27:u16)
  n8 = control-ref of="Data Length 抓資料後的剩餘長度"() -> (w10:refnum<vi>)
  n9 = control-ref of="Data Length 抓資料後的剩餘長度 2"() -> (w9:refnum<vi>)
  n10 = call "TCPIP Connect.vi"("error in (no error)"=w23, "Port"=w24, "TCP address"=w25) -> ("error out"=w8:errorcluster, "CreateIp"=w18:refnum<k24>)  [unwired: 7 in]
  n11 = property class="WFChart (strict)"(reference=w9, "History Data"=w4) -> (error out=w6:errorcluster)  [unwired: 1 in, 1 out]
  n12 = property class="WFChart (strict)"(reference=w10, "History Data"=w4) -> (error out=w7:errorcluster)  [unwired: 1 in, 1 out]
  n13 = Merge Errors(w8, w7, w6) -> (w5:errorcluster)
  n14 = invoke class="ModbusIpMaster" method="ReadHoldingRegisters"(reference=w18, error in=w5, "startAddress"=w47, "numberOfPoints"=u16 1) -> (reference out=w20:refnum<k24>, error out=w19:errorcluster, "ReadHoldingRegisters"=w46:u16[])  [unwired: 1 in, 2 out]
  n15 = Index Array(array=w46) -> (element=→"Device ID":u16)  [unwired: 1 in]
  n16 = invoke class="ModbusIpMaster" method="WriteSingleRegister"(reference=w20, error in=w19, "registerAddress"=w49, "value"=w27) -> (reference out=w40:refnum<k24>, error out=w39:errorcluster)  [unwired: 1 in, 3 out]
  n17 = invoke class="ModbusIpMaster" method="ReadHoldingRegisters"(reference=w40, error in=w39, "startAddress"=w42, "numberOfPoints"=u16 1) -> (reference out=w22:refnum<k24>, error out=w21:errorcluster, "ReadHoldingRegisters"=w38:u16[])  [unwired: 1 in, 2 out]
  n18 = Index Array(array=w38) -> (element=w37:u16)  [unwired: 1 in]
  n19 = Number To Boolean Array(number=w37) -> (Boolean array=w35:bool[])
  n20 = invoke class="ModbusIpMaster" method="WriteSingleRegister"(reference=w22, error in=w21, "registerAddress"=w30, "value"=u16 0) -> (reference out=w29:refnum<k24>, error out=w28:errorcluster)  [unwired: 1 in, 3 out]
  n21 = Split 1D Array(array=w35, index=4) -> (first subarray=w3:bool[], second subarray=→"Failure  (Port1 ~ Port4)":bool[])
  "Connted (Port1 ~ Port4)" <- w3
  n22 = And(x=w3, y="ON (Port1 ~ Port4) 2") -> (x .and. y?=w1:bool[])
  n23 = Index Array(array=w1) -> (element #1=w14:bool, element #2=w13:bool, element #3=w12:bool, element #4=w11:bool)  [unwired: 4 in]
  n24 = Bundle By Name(cluster=w16, "Port1.Connected"=w14, "Port2.Connected"=w13, "Port3.Connected"=w12, "Port4.Connected"=w11) -> (w15:T3)
  n25 = invoke class="ModbusIpMaster" method="WriteSingleRegister"(reference=w29, error in=w28, "registerAddress"=w33, "value"=u16 15) -> (reference out=w43:refnum<k24>, error out=w44:errorcluster)  [unwired: 1 in, 3 out]
  n26 = flat-sequence {
    tunnel: w44 -> [w61]
    tunnel: [w61] -> w54
    frame #0 {
      n27 = Wait (ms)(milliseconds to wait=u32 0) -> ()  [unwired: 1 out]
    }
  }
  n28 = flat-sequence {
    tunnel: [w63] -> w50
    frame #0 {
      n29 = call <vilib>:"Application Directory.vi"() -> ("Application Directory"=w67:path)
      n30 = Build Path(base path=w67, name or relative path="Log") -> (appended path=w65:path)
      n31 = Build Path(base path=w65, name or relative path="bufferSize.txt") -> (appended path=w63:path)
    }
  }
  n32 = Obtain Queue(name (unnamed)="Log", element data type=u16 0 ("Next # 2"), error in (no error)=w54) -> (queue out=w52:refnum<queue>, error out=w53:errorcluster)  [unwired: 2 in, 1 out]
  n33 = while {
    shift-right: [w85] -> w56
    shift-left: w53 -> [w75]
    shift-right: [w82] -> _
    shift-left: w43 -> [w87]
    tunnel: w52 -> [w84]
    tunnel: [w83] -> w51
    tunnel: "Modbus TCP Setting" -> [w72]
    shift-right: [w69] -> _
    shift-left: w15 -> [w71]
    i -> [w86]
    stop <- "stop" stop-if-true
    # "Counter數轉成物理量(g) ,Sensor要與box上的設定一致\n4(g) = 8192\n8(g) = 4096"
    n34 = Unbundle By Name(w72) -> ("CH"=w73:enum16{"Port1", "Port2", "Port3", "Port4"})
    n35 = Unbundle By Name(w75) -> ("code"=w79:i32)
    n36 = case shown="\"Port1\", Default" w73 {
      tunnel: [w96 w97 w98 w99] -> w81
      frame "Port1", Default {
        w96 = u16 0  # CH_Addr
      }
      frame "Port2" {
        w97 = u16 200  # CH_Addr
      }
      frame "Port3" {
        w98 = u16 400  # CH_Addr
      }
      frame "Port4" {
        w99 = u16 600  # CH_Addr
      }
    }
    n37 = Equal?(x=1172, y=w79) -> (x = y?=w77:bool)
    n38 = case shown="False" w77 {
      tunnel: [w88 w91] -> w76
      tunnel: w75 -> [w90 w95]
      tunnel: [w90 w94] -> w74
      tunnel: w71 -> [w89 w93]
      tunnel: [w89 w92] -> w70
      frame False {
        n39 = Unbundle By Name(w89) -> ("ControBoxState"=w88:T1)
      }
      frame True {
        w91 = Modbus_Function_TCP."Recconect Box" ("Modbus Function 2")
        n40 = Bundle By Name(cluster=w93, "ControBoxState"=w91) -> (w92:T3)
        n41 = call <vilib>:"Clear Errors.vi"("error in (no error)"=w95) -> ("error out"=w94:errorcluster)  [unwired: 5 in, 1 out]
      }
    }
    n42 = case shown="\"BoxReady\"" w76 {
      tunnel: w87 -> [w104 w286 _]
      tunnel: [w107 w274 w314] -> w85
      tunnel: [w111 w278 w315] -> w82
      tunnel: w74 -> [w101 w285 w316]
      tunnel: w81 -> [_ _ _]
      tunnel: w73 -> [_ w284 _]
      tunnel: w72 -> [_ _ w319]
      tunnel: w70 -> [w106 w283 w313]
      tunnel: [w108 w276 w312] -> w69
      frame "BoxReady" {
        n43 = Unbundle By Name(w106) -> ("Port2"=w105:T2)
        n44 = Unbundle By Name(w106) -> ("Port1"=w110:T2)
        n45 = flat-sequence {
          tunnel: w104 -> [w199]
          tunnel: [w198] -> w111
          tunnel: w110 -> [w196]
          tunnel: w101 -> [w195]
          tunnel: [w194] -> w109
          tunnel: [w193] -> w100
          frame #0 {
            n46 = Unbundle By Name(w196) -> ("Connected"=w197:bool)
            n47 = case shown="True" w197 {
              tunnel: w199 -> [w202 w226]
              tunnel: [w202 w225] -> w198
              tunnel: w196 -> [w201 w220]
              tunnel: w195 -> [w200 w222]
              tunnel: [w201 w219] -> w194
              tunnel: [w200 w218] -> w193
              frame False {
              }
              frame True {
                w207 = 8192 ("length")
                n48 = Unbundle By Name(w220) -> ("PortOffset_Addr"=w203:u16, "# samplesRVTbuffer"=w224:u16)
                n49 = call "Check data length_PortX.vi"("error in"=w222, "# samples in buffer"=w224) -> ("error iout"=w221:errorcluster, "Modbus Function"=w217:T1, "# samples in buffer out"=w223:u16)  [unwired: 7 in]
                n50 = case shown="\"Normal Mode\", Default" w217 {
                  tunnel: w226 -> [w232 w249 w271]
                  tunnel: [w234 w253 w267] -> w204
                  tunnel: [w236 w251 w269] -> w218
                  tunnel: [w233 w248 w270] -> w225
                  tunnel: w221 -> [w237 w250 w272]
                  tunnel: [w235 w252 _] -> w205
                  tunnel: w223 -> [w229 w247 _]
                  tunnel: w203 -> [w227 w245 w264]
                  frame "Normal Mode", Default {
                    w242 = u16 2  # Data Length + Rawdata
                    # "Normal Mode"
                    n51 = In Range and Coerce(upper limit=u16 123, x=w229, lower limit=u16 0) -> (coerced(x)=w238:u16)  [unwired: 1 out]
                    n52 = Increment(x=w238) -> (x+1=w231:u16)
                    n53 = Add(x=w227, y=w242) -> (x+y=w228:u16)
                    n54 = invoke class="ModbusIpMaster" method="ReadInputRegisters"(reference=w232, error in=w237, "startAddress"=w228, "numberOfPoints"=w231) -> (reference out=w233:refnum<k24>, error out=w236:errorcluster, "ReadInputRegisters"=w230:u16[])  [unwired: 1 in, 2 out]
                    n55 = Delete From Array(array=w230, length=1, index=0) -> (deleted portion=w241:u16[], array with subset deleted=w235:u16[])
                    n56 = Index Array(array=w241) -> (element=w234:u16)  [unwired: 1 in]
                  }
                  frame "Bulk Mode" {
                    w262 = u16 21  # #Remaining + Rawdata
                    n57 = Increment(x=w247) -> (x+1=w256:u16)
                    n58 = Replace Array Subset(array=u16[] [0], new element=w256, index=0) -> (w260:u16[])
                    n59 = Add(x=w245, y=w262) -> (x+y=w246:u16)
                    n60 = invoke class="ModbusIpMaster" method="ReadBulkRegisters"(reference=w249, error in=w250, "startAddress"=w246, "max_size"=i16 9, "Vib_dat"=w260) -> (reference out=w248:refnum<k24>, error out=w251:errorcluster, "Vib_dat"=w263:u16[])  [unwired: 1 in, 3 out]
                    n61 = Delete From Array(array=w263, length=1, index=0) -> (deleted portion=w259:u16[], array with subset deleted=w252:u16[])
                    n62 = Index Array(array=w259) -> (element=w253:u16)  [unwired: 1 in]
                  }
                  frame "Get Data Length" {
                    w273 = u16 2  # Data Length + Rawdata
                    n63 = Add(x=w264, y=w273) -> (x+y=w265:u16)
                    n64 = invoke class="ModbusIpMaster" method="ReadInputRegisters"(reference=w271, error in=w272, "startAddress"=w265, "numberOfPoints"=u16 1) -> (reference out=w270:refnum<k24>, error out=w269:errorcluster, "ReadInputRegisters"=w268:u16[])  [unwired: 1 in, 2 out]
                    n65 = Index Array(array=w268) -> (element=w267:u16)  [unwired: 1 in]
                  }
                }
                "Data Length 抓資料後的剩餘長度" <- w204
                n66 = Bundle By Name(cluster=w220, "# samplesRVTbuffer"=w204, "State"=w217) -> (w219:T2)
                n67 = Type Cast(type=i16[] [], x=w205) -> (*(type *) &x=w216:i16[])
                n68 = Decimate 1D Array(w216) -> (w215:i16[], w214:i16[], w213:i16[])
                n69 = Divide(x=w215, y=w207) -> (x/y=w212:dbl[])
                n70 = Divide(x=w214, y=w207) -> (x/y=w211:dbl[])
                n71 = Divide(x=w213, y=w207) -> (x/y=w210:dbl[])
                n72 = Build Array(w212, w211, w210) -> (w209:dbl[][])
                n73 = Transpose 2D Array(2D array=w209) -> (transposed array=→"Waveform Chart":dbl[][])
              }
            }
          }
        }
        n74 = flat-sequence {
          tunnel: w104 -> [w118]
          tunnel: [w117] -> _
          tunnel: w105 -> [w115]
          tunnel: w100 -> [w114]
          tunnel: [w113] -> w103
          tunnel: [w112] -> w102
          frame #0 {
            n75 = Unbundle By Name(w115) -> ("Connected"=w116:bool)
            n76 = case shown="True" w116 {
              tunnel: w118 -> [w121 w145]
              tunnel: [w121 w144] -> w117
              tunnel: w115 -> [w120 w139]
              tunnel: w114 -> [w119 w141]
              tunnel: [w120 w138] -> w113
              tunnel: [w119 w137] -> w112
              frame False {
              }
              frame True {
                w126 = 8192 ("length")
                n77 = Unbundle By Name(w139) -> ("PortOffset_Addr"=w122:u16, "# samplesRVTbuffer"=w143:u16)
                n78 = call "Check data length_PortX.vi"("error in"=w141, "# samples in buffer"=w143) -> ("error iout"=w140:errorcluster, "Modbus Function"=w136:T1, "# samples in buffer out"=w142:u16)  [unwired: 7 in]
                n79 = case shown="\"Normal Mode\", Default" w136 {
                  tunnel: w145 -> [w151 w168 w190]
                  tunnel: [w153 w172 w186] -> w123
                  tunnel: [w155 w170 w188] -> w137
                  tunnel: [w152 w167 w189] -> w144
                  tunnel: w140 -> [w156 w169 w191]
                  tunnel: [w154 w171 _] -> w124
                  tunnel: w142 -> [w148 w166 _]
                  tunnel: w122 -> [w146 w164 w183]
                  frame "Normal Mode", Default {
                    w161 = u16 2  # Data Length + Rawdata
                    # "Normal Mode"
                    n80 = In Range and Coerce(upper limit=u16 123, x=w148, lower limit=u16 0) -> (coerced(x)=w157:u16)  [unwired: 1 out]
                    n81 = Increment(x=w157) -> (x+1=w150:u16)
                    n82 = Add(x=w146, y=w161) -> (x+y=w147:u16)
                    n83 = invoke class="ModbusIpMaster" method="ReadInputRegisters"(reference=w151, error in=w156, "startAddress"=w147, "numberOfPoints"=w150) -> (reference out=w152:refnum<k24>, error out=w155:errorcluster, "ReadInputRegisters"=w149:u16[])  [unwired: 1 in, 2 out]
                    n84 = Delete From Array(array=w149, length=1, index=0) -> (deleted portion=w160:u16[], array with subset deleted=w154:u16[])
                    n85 = Index Array(array=w160) -> (element=w153:u16)  [unwired: 1 in]
                  }
                  frame "Bulk Mode" {
                    w181 = u16 21  # #Remaining + Rawdata
                    n86 = Increment(x=w166) -> (x+1=w175:u16)
                    n87 = Replace Array Subset(array=u16[] [0], new element=w175, index=0) -> (w179:u16[])
                    n88 = Add(x=w164, y=w181) -> (x+y=w165:u16)
                    n89 = invoke class="ModbusIpMaster" method="ReadBulkRegisters"(reference=w168, error in=w169, "startAddress"=w165, "max_size"=i16 9, "Vib_dat"=w179) -> (reference out=w167:refnum<k24>, error out=w170:errorcluster, "Vib_dat"=w182:u16[])  [unwired: 1 in, 3 out]
                    n90 = Delete From Array(array=w182, length=1, index=0) -> (deleted portion=w178:u16[], array with subset deleted=w171:u16[])
                    n91 = Index Array(array=w178) -> (element=w172:u16)  [unwired: 1 in]
                  }
                  frame "Get Data Length" {
                    w192 = u16 2  # Data Length + Rawdata
                    n92 = Add(x=w183, y=w192) -> (x+y=w184:u16)
                    n93 = invoke class="ModbusIpMaster" method="ReadInputRegisters"(reference=w190, error in=w191, "startAddress"=w184, "numberOfPoints"=u16 1) -> (reference out=w189:refnum<k24>, error out=w188:errorcluster, "ReadInputRegisters"=w187:u16[])  [unwired: 1 in, 2 out]
                    n94 = Index Array(array=w187) -> (element=w186:u16)  [unwired: 1 in]
                  }
                }
                "Data Length 抓資料後的剩餘長度 2" <- w123
                n95 = Bundle By Name(cluster=w139, "# samplesRVTbuffer"=w123, "State"=w136) -> (w138:T2)
                n96 = Type Cast(type=i16[] [], x=w124) -> (*(type *) &x=w135:i16[])
                n97 = Decimate 1D Array(w135) -> (w134:i16[], w133:i16[], w132:i16[])
                n98 = Divide(x=w134, y=w126) -> (x/y=w131:dbl[])
                n99 = Divide(x=w133, y=w126) -> (x/y=w130:dbl[])
                n100 = Divide(x=w132, y=w126) -> (x/y=w129:dbl[])
                n101 = Build Array(w131, w130, w129) -> (w128:dbl[][])
                n102 = Transpose 2D Array(2D array=w128) -> (transposed array=→"Waveform Chart 2":dbl[][])
              }
            }
          }
        }
        n103 = Bundle By Name(cluster=w106, "Port1"=w109, "Port2"=w103) -> (w108:T3)
        n104 = Merge Errors(w100, w102) -> (w107:errorcluster)
      }
      frame "Reconnect Port" {
        w275 = u16 0 ("Port1.# samplesRVTbuffer")
        w281 = u16 22  # ClearPortBuffer
        # "ALL PORT"
        n105 = while {
          tunnel: w286 -> [w305]
          tunnel: w285 -> [w304]
          tunnel: w284 -> [w296]
          tunnel: [w289] -> w279
          tunnel: [w293] -> w280
          tunnel: w283 -> [w288]
          tunnel: [w287] -> w277
          stop <- w295 stop-if-true
          w299 = u16 13  # Sensor State
          w307 = u16 2023  # Sensor  Reconnect
          # "Recconect Sensor per 0.5 s"
          n106 = invoke class="ModbusIpMaster" method="WriteSingleRegister"(reference=w305, error in=w304, "registerAddress"=w307, "value"=u16 1) -> (reference out=w297:refnum<k24>, error out=w291:errorcluster)  [unwired: 1 in, 3 out]
          n107 = call "Time Delay"("error in (no error)"=w291, "Delay Time (s)"=0.5) -> ("error out"=w290:errorcluster)  [unwired: 9 in]
          n108 = invoke class="ModbusIpMaster" method="ReadHoldingRegisters"(reference=w297, error in=w290, "startAddress"=w299, "numberOfPoints"=u16 1) -> (reference out=w293:refnum<k24>, error out=w289:errorcluster, "ReadHoldingRegisters"=w302:u16[])  [unwired: 1 in, 2 out]
          n109 = Index Array(array=w302) -> (element=w301:u16)  [unwired: 1 in]
          n110 = case shown="No Error" w289 {
            tunnel: [w310 w311] -> w287
            tunnel: w288 -> [w308 w311]
            frame No Error {
              n111 = Bundle By Name(cluster=w308, "ControBoxState"=Modbus_Function_TCP."BoxReady") -> (w310:T3)
            }
            frame Error {
            }
          }
          n112 = Number To Boolean Array(number=w301) -> (Boolean array=w300:bool[])
          n113 = Split 1D Array(array=w300, index=4) -> (first subarray=w303:bool[])  [unwired: 1 out]
          n114 = Index Array(array=w303, index=w296) -> (element=w295:bool)
        }
        n115 = Bundle By Name(cluster=w277, "Port1.# samplesRVTbuffer"=w275, "Port2.# samplesRVTbuffer"=w275, "Port3.# samplesRVTbuffer"=w275, "Port4.# samplesRVTbuffer"=w275) -> (w276:T3)
        n116 = invoke class="ModbusIpMaster" method="WriteSingleRegister"(reference=w280, error in=w279, "registerAddress"=w281, "value"=u16 15) -> (reference out=w278:refnum<k24>, error out=w274:errorcluster)  [unwired: 1 in, 3 out]
      }
      frame "Recconect Box", Default {
        n117 = Unbundle By Name(w319) -> ("TCP address"=w318:string, "Port"=w317:i32)
        n118 = call "TCPIP Connect.vi"("error in (no error)"=w316, "Port"=w317, "TCP address"=w318) -> ("error out"=w314:errorcluster, "CreateIp"=w315:refnum<k24>)  [unwired: 7 in]
        n119 = case shown="No Error" w314 {
          tunnel: w313 -> [w322 w323]
          tunnel: [w321 w323] -> w312
          frame No Error {
            n120 = Bundle By Name(cluster=w322, "ControBoxState"=Modbus_Function_TCP."Reconnect Port") -> (w321:T3)
          }
          frame Error {
          }
        }
      }
    }
    "State" <- w69
    n121 = Unbundle By Name(w69) -> ("Port1.# samplesRVTbuffer"=w68:u16)
    "Next #" <- w68
    n122 = Enqueue Element(queue=w84, element=w68) -> (queue out=w83:refnum<queue>)  [unwired: 2 in, 2 out]
    "Iteration" <- w86
  }
  n123 = while {
    tunnel: w52 -> [w333]
    shift-right: [w329] -> _
    shift-left: w53 -> [w334]
    tunnel: w50 -> [w328]
    stop <- w331 stop-if-true
    n124 = Dequeue Element(queue=w333, error in (no error)=w334) -> (element=w327:u16, error out=w330:errorcluster)  [unwired: 1 in, 2 out]
    n125 = Get Date/Time In Seconds() -> (seconds since 1Jan1904=w326:timestamp)
    n126 = Format Date/Time String(time format string (%c)="%Y/%m/%d %H:%M:%S%3u", seconds (now)=w326) -> (date/time string=w325:string)  [unwired: 1 in]
    n127 = call "Write To Measurement File"("Signals"=w327, "error in (no error)"=w330, "Filename"=w328, "Comment"=w325) -> ("error out"=w329:errorcluster)  [unwired: 13 in, 2 out]
    n128 = local read "stop"() -> (w332:bool)
    n129 = Or(x=w329, y=w332) -> (x .or. y?=w331:bool)
  }
  n130 = flat-sequence {
    tunnel: w56 -> [w337]
    tunnel: w51 -> [w335]
    frame #0 {
      n131 = Release Queue(queue=w335, error in (no error)=w337) -> (error out=→"error out":errorcluster)  [unwired: 1 in, 2 out]
      n132 = Get Date/Time In Seconds() -> (seconds since 1Jan1904=→"Stop Time":timestamp)
    }
  }
